vi "MSScript_Format_ResetRFPhase.vi"(9 "ValueArray":string[](array[string]), 10 "TagArray":string[](array[string]), 11 "MSScript.lvclass":refnum<class "MSScript.lvclass">) -> (0 "ValueErrorArray":bool[](array[boolean]), 1 "TagErrorArray":bool[](array[boolean]), 2 "ParamErrorArray":bool[](array[boolean]), 3 "Data":variant, 4 "#ofParamError":bool)   [LabVIEW 2018, in "MSScript.lvclass"]
uses:
  MSScript.lvclass
  Ctl/MSEditorParam resetRFCycle.ctl
  MSScript_Transform_UInt.vi
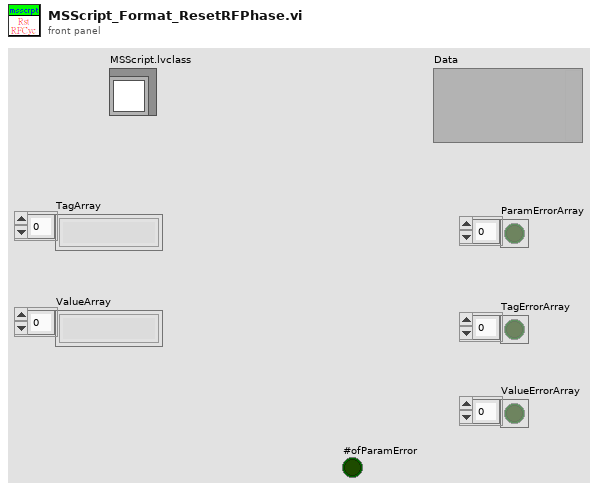
[diagram p1: front panel]
types:
  T1 = typedef "MSEditorParam resetRFCycle.ctl" = cluster{"iniPhase":u32}
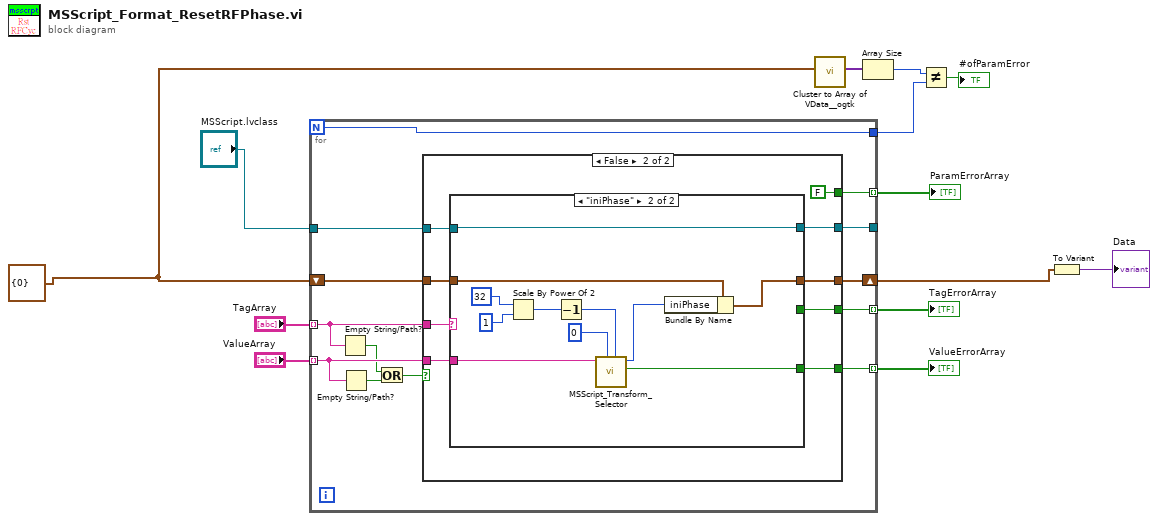
[diagram p0: block diagram]
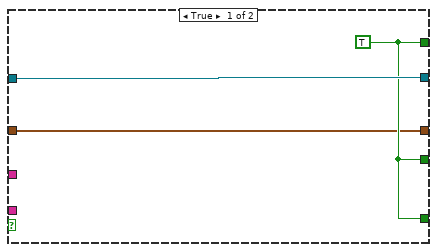
[diagram p2: hidden frame]
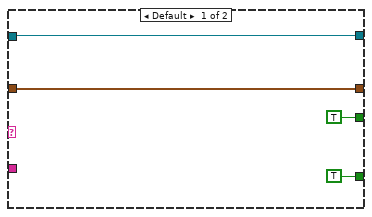
[diagram p3: hidden frame]
diagram:
  w1 = T1 {"iniPhase"=0} ("ParamValueType")
  n1 = for {
    N -> [w14]
    tunnel: "TagArray" -> [w22] mode=indexing
    tunnel: "ValueArray" -> [w21] mode=indexing
    tunnel: [w26] -> w11 mode=indexing
    tunnel: "MSScript.lvclass" -> [w25]
    tunnel: [w24] -> w10 mode=indexing
    tunnel: [w23] -> _
    tunnel: [w17] -> w9 mode=indexing
    shift-right: [w15] -> w3
    shift-left: w1 -> [w16]
    tunnel: [w14] -> w4
    n2 = Empty String/Path?(string/path=w22) -> (empty?=w19:bool)
    n3 = Empty String/Path?(string/path=w21) -> (empty?=w20:bool)
    n4 = Or(x=w19, y=w20) -> (x .or. y?=w18:bool)
    n5 = case shown="False" w18 {
      tunnel: [w28 w31] -> w26
      tunnel: w25 -> [w29 w34]
      tunnel: [w28 w30] -> w24
      tunnel: [w29 w33] -> w23
      tunnel: w22 -> [_ w36]
      tunnel: w21 -> [_ w37]
      tunnel: [w28 FALSE] -> w17
      tunnel: w16 -> [w27 w35]
      tunnel: [w27 w32] -> w15
      frame True {
        w28 = TRUE
      }
      frame False {
        n6 = case shown="\"iniPhase\"" w36 {
          tunnel: [TRUE _] -> w31
          tunnel: w37 -> [_ w52]
          tunnel: [TRUE ("Value Error?") w53] -> w30
          tunnel: [w40 w49] -> w33
          tunnel: [w39 w51] -> w32
          tunnel: w35 -> [w39 w50]
          tunnel: w34 -> [w40 w49]
          frame Default {
          }
          frame "iniPhase" {
            n7 = Scale By Power Of 2(n=i16 32, x=u64 1 ("upper limit")) -> (x*2^n=w44:u64)
            n8 = Decrement(x=w44) -> (x-1=w43:u64)
            n9 = call-poly "MSScript_Transform_Selector.vi"("upper limit"=w43, "lower limit"=u64 0 ("upper limit"), "string in"=w52) -> ("Value Error?"=w53:bool, "Value Output"=w47:u64)  [unwired: 6 in, 1 out]
            n10 = Bundle By Name(cluster=w50, "iniPhase"=w47) -> (w51:T1)
          }
        }
      }
    }
  }
  "TagErrorArray" <- w11
  "ValueErrorArray" <- w10
  "ParamErrorArray" <- w9
  n11 = call <userlib>:"Cluster to Array of VData__ogtk.vi"("Cluster"=w1) -> ("Array of VData"=w7:variant[])  [unwired: 9 in, 1 out]
  n12 = Array Size(array=w7) -> (size(s)=w6:i32)
  n13 = Not Equal?(x=w6, y=w4) -> (x != y?=→"#ofParamError":bool)
  n14 = To Variant(anything=w3) -> (Variant=→"Data":variant)
